vi "RequestActiveAlarms.vi"(8 "error in (no error)":errorcluster, 10 "Qbus in":refnum<class "Qbus.lvclass">, 11 "config":T1) -> (0 "error out":errorcluster)   [LabVIEW 2017, in "TrendAlarm.lvlib"]
uses:
  <vilib>/addons/InsightCM/Devices/Shared/Common/TrendAlarm/TrendAlarm.lvlib
  <vilib>/addons/InsightCM/Devices/Shared/Common/TrendAlarm/controls/config.ctl
  <vilib>/addons/Qbus/Qbus.lvclass
  <vilib>/addons/InsightCM/MessageBus/MessageLibrary/TrendAlarm/controls/AlarmQueryActiveTrendInstancesRequestBody.ctl
  <vilib>/addons/InsightCM/Devices/Shared/Common/ServerComm/ServerComm.lvlib
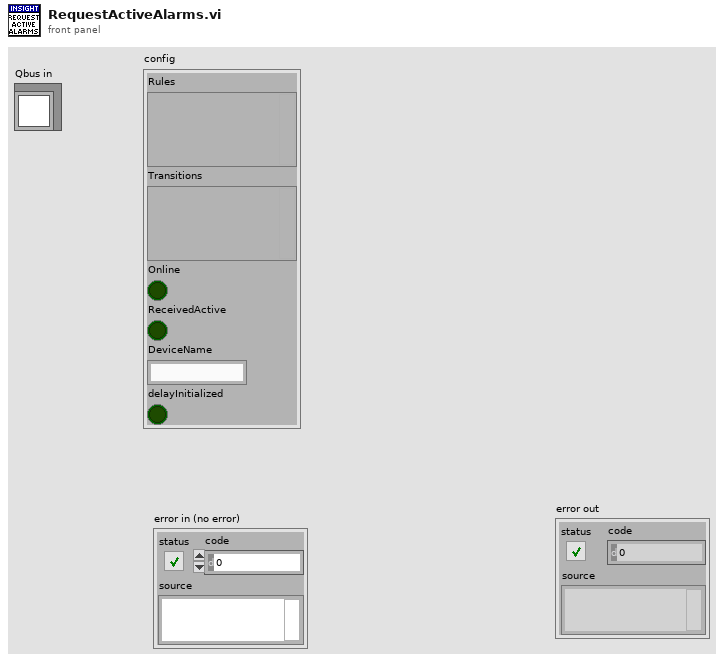
[diagram p1: front panel]
types:
  T1 = typedef "TrendAlarm.lvlib/config.ctl" = cluster{"Rules":variant, "Transitions":variant, "Online":bool, "ReceivedActive":bool, "DeviceName":string, "delayInitialized":bool}
  T2 = typedef "AlarmQueryActiveTrendInstancesRequestBody.ctl" = cluster{"RuleIds":string[], "Skip":i32, "Take":i32}
  T3 = typedef "Message.ctl" = cluster{"Header":T4, "Body":u8[]}
  T4 = typedef "MessageHeader.ctl" = cluster{"MessageName":string, "Timestamp":i64, "CorrelationId":string, "ContentType":string, "RoutingKey":string, "Properties":T5[]}
  T5 = typedef "KeyValuePair.ctl" = cluster{"Key":string, "Value":string}
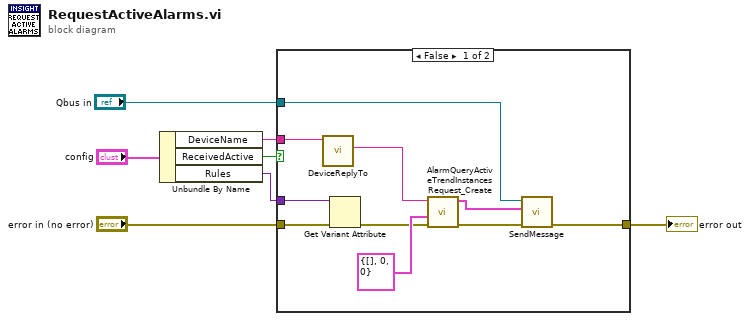
[diagram p0: block diagram]
diagram:
  n1 = Unbundle By Name("config") -> ("DeviceName"=w3:string, "ReceivedActive"=w6:bool, "Rules"=w4:variant)
  n2 = case shown="False" w6 {
    tunnel: "error in (no error)" -> [w17 w18]
    tunnel: w4 -> [w16 _]
    tunnel: w3 -> [w15 _]
    tunnel: [w14 w18] -> w2
    tunnel: "Qbus in" -> [w13 _]
    frame False {
      n3 = call <vilib>:"DeviceReplyTo.vi"("Device"=w15) -> ("ReplyTo"=w12:string)  [unwired: 10 in]
      n4 = Get Variant Attribute(Variant=w16, error in=w17) -> (error out=w10:errorcluster)  [unwired: 2 in, 3 out]
      n5 = call <vilib>:"AlarmQueryActiveTrendInstancesRequest_Create.vi"("error in (no error)"=w10, "AlarmQueryActiveTrendInstancesRequest"=T2 {"RuleIds"=[], "Skip"=0, "Take"=0}, "ReplyTo"=w12) -> ("error out"=w8:errorcluster, "Message"=w9:T3)  [unwired: 7 in]
      n6 = call <vilib>:"SendMessage.vi"("error in (no error)"=w8, "message"=w9, "Qbus in"=w13) -> ("error out"=w14:errorcluster)  [unwired: 7 in, 1 out]
    }
    frame True {
    }
  }
  "error out" <- w2
